vi "LVIS_IsGlobal.vi"() -> ()   [LabVIEW 2015]
panel:
  out "Status":T1
  in  "CfgEventInfo":T2={"EventName"="*", "EventStart"="*", "EventStop"="*", "EventStatus"="*", "EventClientID"="*", "IS_EventID"="*", "EventMeta"="*", "ProductLine"="*", "ProcessName"="*", "Station"="*", "Operator"="*", "SN"="*", "Model"="*", "Manufacturer"="*"}
  in  "Station":string
  in  "LibPath":path
  in  "EventData":T3(array[cluster])
  out "CustomError":cluster{"Code":i32, "Source":string}[](array[cluster])=[{"Code"=5000, "Source"="Data field [EventName] is blank."}, {"Code"=5001, "Source"="Data field [EventName] does not end in (_Event)."}, {"Code"=5002, "Source"="Data field [EventStart] is blank."}, {"Code"=5003, "Source"="Data field [EventStop] is blank."}, {"Code"=5004, "Source"="Data field [EventStatus] is blank."}, {"Code"=5005, "Source"="Data field [EventStatus] does not contain an accepted value."}, {"Code"=5006, "Source"="Data field [EventClientIS] is blank."}, {"Code"=5007, "Source"="Data field [IS_EventID] is blank."}, {"Code"=5008, "Source"="Data field [IS_EventID] does not equal (-1)."}, {"Code"=5009, "Source"="Data field [ProductLine] does not contain an accepted value."}, {"Code"=5010, "Source"="Data field [ProcessName] is blank."}, {"Code"=5011, "Source"="Data field [ProcessName] does not contain an accepted value."}, {"Code"=5012, "Source"="Data field [Station] is blank."}, {"Code"=5013, "Source"="Data field [Operator] is blank."}, {"Code"=5014, "Source"="Data field [SN] is blank."}, {"Code"=5015, "Source"="Data field [Model] is blank."}, {"Code"=5016, "Source"="Data field [Manufacturer] is blank."}, {"Code"=5017, "Source"="Data field [Manufacturer] does not contain an accepted value."}, {"Code"=5030, "Source"="Data field [TestName] is blank."}, {"Code"=5031, "Source"="Data field [TestName] does not end in (_Tests)."}, {"Code"=5032, "Source"="Data field [TestDateTime] is blank."}, {"Code"=5033, "Source"="Data field [TestStatus] is blank."}, {"Code"=5034, "Source"="Data field [TestStatus] does not contain an accepted value."}, {"Code"=5035, "Source"="Data field [TestClientID] is blank."}, {"Code"=5036, "Source"="Data field [IS_TestID] is blank."}, {"Code"=5037, "Source"="Data field [IS_TestID] does not equal (-1)."}, {"Code"=5050, "Source"="Data field [MeasName] is blank."}, {"Code"=5051, "Source"="Data field [MeasDateTime] is blank."}, {"Code"=5052, "Source"="Data field [MeasStatus] is blank."}, {"Code"=5053, "Source"="Data field [MeasStatus] does not contain an accepted value."}, {"Code"=5054, "Source"="Data field [MeasClientID] is blank."}, {"Code"=5055, "Source"="Data field [IS_MeasID] is blank."}, {"Code"=5056, "Source"="Data field [IS_MeasID] does not equal (-1)."}, {"Code"=5057, "Source"="Data field [MeasType] is blank."}, {"Code"=5058, "Source"="Data field [MeasType] does not contain an accepted value."}, {"Code"=5059, "Source"="Data field [LL] is blank."}, {"Code"=5060, "Source"="Data field [LL Comp] is blank."}, {"Code"=5061, "Source"="Data field [LL Comp] does not contain an accepted value."}, {"Code"=5062, "Source"="Data field [HL] is blank."}, {"Code"=5063, "Source"="Data field [HL Comp] is blank."}, {"Code"=5064, "Source"="Data field [HL Comp] does not contain an accepted value."}, {"Code"=5075, "Source"="Data field string length is too long."}, {"Code"=5100, "Source"="The Data Commander Sent and Received CRCs don't match."}, {"Code"=5101, "Source"="The Data Commander Errror Count field is not zero."}, {"Code"=5102, "Source"="The Data Commander returned a non-zero status."}, {"Code"=5103, "Source"="The Data Commander did not respond to a ping request."}, {"Code"=5150, "Source"="Invalid combination of \"LastTestMeas?\" and \"LastEventMeas?\" controls."}]
  in  "EventInfo":T2={"EventName"="*", "EventStart"="*", "EventStop"="*", "EventStatus"="*", "EventClientID"="*", "IS_EventID"="*", "EventMeta"="", "ProductLine"="*", "ProcessName"="*", "Station"="*", "Operator"="*", "SN"="*", "Model"="*", "Manufacturer"="*"}
  in  "TestData":string[][][](array[string])
  in  "MeasInfo":T4
  in  "TestInfo":T5
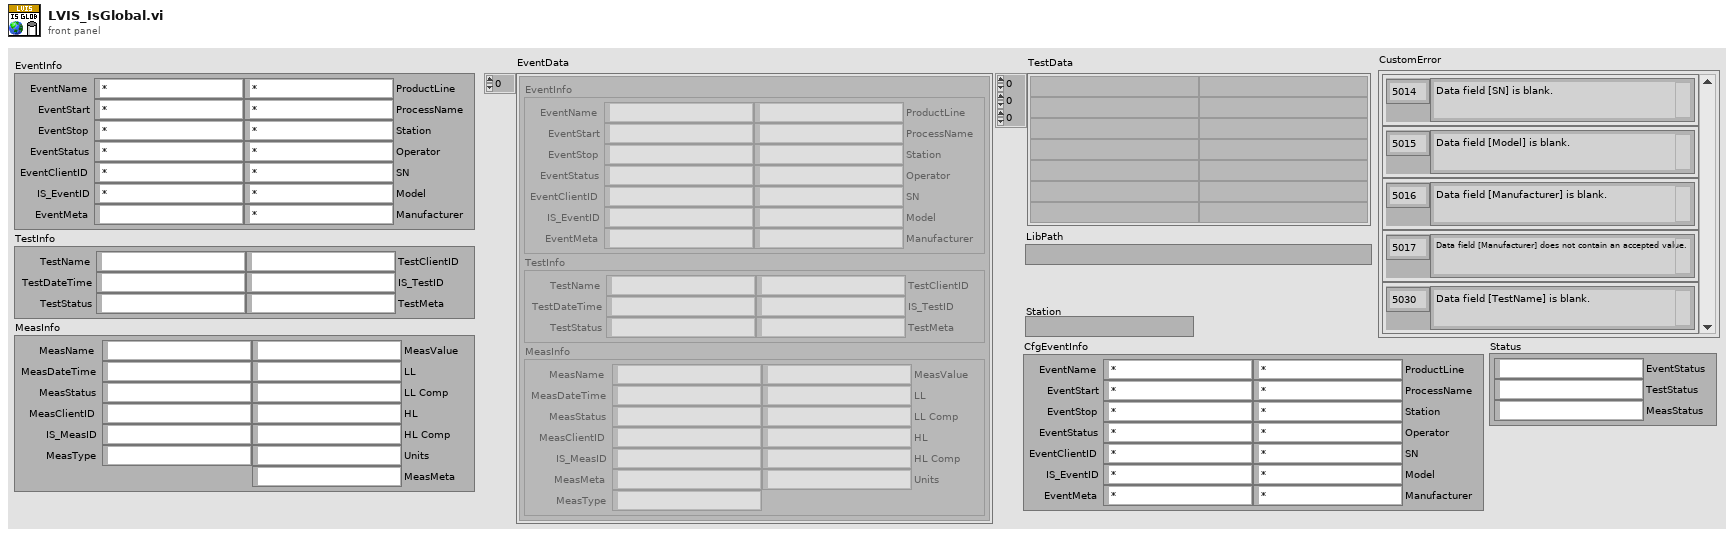
[diagram p1: front panel]
types:
  T1 = cluster{"EventStatus":string, "TestStatus":string, "MeasStatus":string}
  T2 = cluster{"EventName":string, "EventStart":string, "EventStop":string, "EventStatus":string, "EventClientID":string, "IS_EventID":string, "EventMeta":string, "ProductLine":string, "ProcessName":string, "Station":string, "Operator":string, "SN":string, "Model":string, "Manufacturer":string}
  T3 = cluster{"EventInfo":cluster{"EventName":string, "EventStart":string, "EventStop":string, "EventStatus":string, "EventClientID":string, "IS_EventID":string, "EventMeta":string, "ProductLine":string, "ProcessName":string, "Station":string, "Operator":string, "SN":string, "Model":string, "Manufacturer":string}, "TestInfo":cluster{"TestName":string, "TestDateTime":string, "TestStatus":string, "TestClientID":string, "IS_TestID":string, "TestMeta":string}, "MeasInfo":cluster{"MeasName":string, "MeasDateTime":string, "MeasStatus":string, "MeasClientID":string, "IS_MeasID":string, "MeasMeta":string, "MeasType":string, "MeasValue":string, "LL":string, "LL Comp":string, "HL":string, "HL Comp":string, "Units":string}}[]
  T4 = cluster{"MeasName":string, "MeasDateTime":string, "MeasStatus":string, "MeasClientID":string, "IS_MeasID":string, "MeasType":string, "MeasValue":string, "LL":string, "LL Comp":string, "HL":string, "HL Comp":string, "Units":string, "MeasMeta":string}
  T5 = cluster{"TestName":string, "TestDateTime":string, "TestStatus":string, "TestClientID":string, "IS_TestID":string, "TestMeta":string}
diagram:
